vi "Initialize Graph.vi"(8 "error in":errorcluster, 11 "WaveformGraph":refnum<vi>) -> (0 "error out":errorcluster)   [LabVIEW 2020, in "TdmsFileViewer.lvlib"]
uses:
  TdmsFileViewer.lvlib
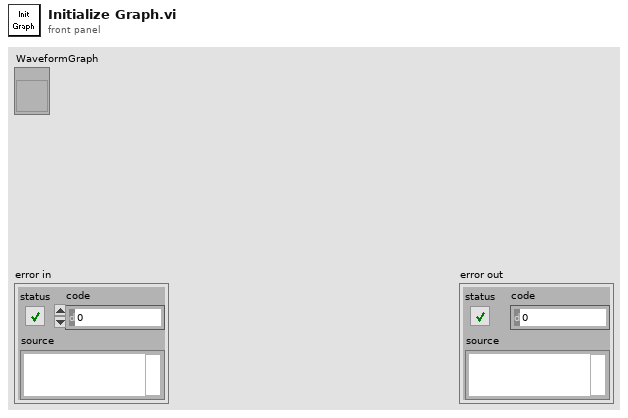
[diagram p1: front panel]
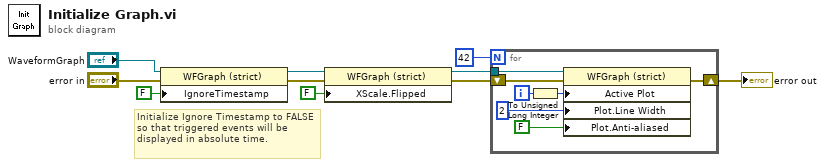
[diagram p0: block diagram]
diagram:
  # "Initialize Ignore Timestamp to FALSE so that triggered events will be displayed in absolute time."
  n1 = property class="WFGraph (strict)"(reference="WaveformGraph", error in="error in", "IgnoreTimestamp"=FALSE ("Ignore Timestamp")) -> (reference out=w5:refnum<vi>, error out=w4:errorcluster)
  n2 = property class="WFGraph (strict)"(reference=w5, error in=w4, "XScale.Flipped"=FALSE ("X Scale.Flipped")) -> (reference out=w3:refnum<vi>, error out=w2:errorcluster)
  n3 = for {
    N: 42 -> [_]
    tunnel: w3 -> [w15]
    shift-right: [w16] -> w10
    shift-left: w2 -> [w17]
    i -> [w11]
    n4 = To Unsigned Long Integer(number=w11) -> (unsigned 32bit integer=w13:u32)
    n5 = property on="Property Node" class="WFGraph (strict)"(reference=w15, error in=w17, "Active Plot"=w13, "Plot.Line Width"=u8 2, "Plot.Anti-aliased"=FALSE) -> (error out=w16:errorcluster)  [unwired: 1 out]
  }
  "error out" <- w10
